vi "Wfm rozszerz do okna.vi"(6 "Wykresy Edit":i32=1290, 8 "error in (no error)":errorcluster, 11 "Wfm Refs in":refnum<vi>[](array[refnum])) -> (0 "error out":errorcluster, 3 "Wfm Refs out":refnum<vi>[](array[refnum]))   [LabVIEW 2014]
doc: "rozszerza szerokoœæ wykresów do okna"
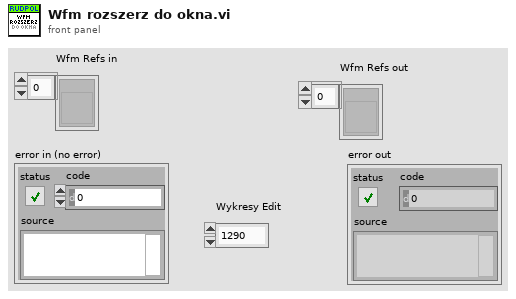
[diagram p1: front panel]
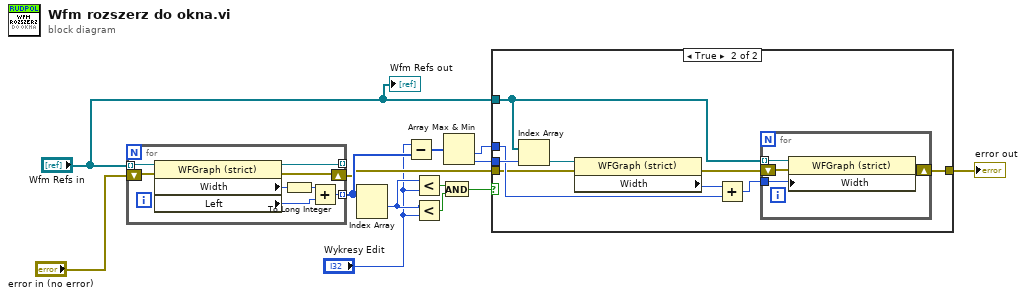
[diagram p0: block diagram]
diagram:
  n1 = for {
    tunnel: "Wfm Refs in" -> [w21] mode=indexing
    shift-right: [w19] -> w4
    shift-left: "error in (no error)" -> [w20]
    tunnel: [w15] -> w9 mode=indexing
    tunnel: [w14] -> _ mode=indexing
    n2 = property class="WFGraph (strict)"(reference=w21, error in=w20) -> (reference out=w14:refnum<vi>, error out=w19:errorcluster, "Width"=w18:u32, "Left"=w16:i32)
    n3 = To Long Integer(number=w18) -> (32bit integer=w17:i32)
    n4 = Add(x=w17, y=w16) -> (x+y=w15:i32)
  }
  n5 = Index Array(array=w9) -> (element #1=w6:i32)  [unwired: 2 in, 1 out]
  n6 = Subtract(x="Wykresy Edit", y=w9) -> (x-y=w10:i32[])
  n7 = Less?(x=w6, y="Wykresy Edit") -> (x < y?=w8:bool)
  n8 = Less?(x=w6, y="Wykresy Edit") -> (x < y?=w7:bool)
  n9 = And(x=w8, y=w7) -> (x .and. y?=w11:bool)
  n10 = Array Max & Min(array=w10) -> (min value=w13:i32, min index (indices)=w12:i32)  [unwired: 2 out]
  n11 = case shown="True" w11 {
    tunnel: w12 -> [_ w30]
    tunnel: w13 -> [_ w28]
    tunnel: "Wfm Refs in" -> [_ w27]
    tunnel: w4 -> [w22 w25]
    tunnel: [w22 w23] -> w2
    frame False {
    }
    frame True {
      n12 = Index Array(array=w27, index=w30) -> (element=w31:refnum<vi>)
      n13 = property class="WFGraph (strict)"(reference=w31, error in=w25) -> (error out=w24:errorcluster, "Width"=w29:u32)  [unwired: 1 out]
      n14 = Add(x=w29, y=w28) -> (x+y=w26:u32)
      n15 = for {
        shift-right: [w34] -> w23
        shift-left: w24 -> [w35]
        tunnel: w27 -> [w33] mode=indexing
        tunnel: w26 -> [w32]
        n16 = property class="WFGraph (strict)"(reference=w33, error in=w35, "Width"=w32) -> (error out=w34:errorcluster)  [unwired: 1 out]
      }
    }
  }
  "error out" <- w2
  "Wfm Refs out" <- "Wfm Refs in"
